vi "test-create-path-trajectory-2.vi"() -> ()   [LabVIEW 2019]
uses:
  <vilib>/Rock Robotics/WPI/ThirdParty/MJansen/PathPlanner/TypeDef/PathPlannerTrajectory.ctl
  <vilib>/Rock Robotics/WPI/ThirdParty/MJansen/PathPlanner/TypeDef/PathPlannerTrajectoryState.ctl
  <vilib>/Rock Robotics/WPI/ThirdParty/JAS_Junk/TrajLib/TypeDef/TRANSLATION2D.ctl
  <vilib>/Rock Robotics/WPI/ThirdParty/JAS_Junk/TrajLib/TypeDef/ROTATION2D.ctl
  <vilib>/Rock Robotics/WPI/ThirdParty/MJansen/PathPlanner/TypeDef/PathPlannerPathConstraints.ctl
  <vilib>/Rock Robotics/WPI/ThirdParty/JAS_Junk/TrajLib/TypeDef/TRAJ_STATE.ctl
  <vilib>/Rock Robotics/WPI/ThirdParty/JAS_Junk/TrajLib/TypeDef/POSE2D.ctl
  <vilib>/Rock Robotics/WPI/ThirdParty/JAS_Junk/TrajLib/TypeDef/CHASSIS_SPEEDS.ctl
  <vilib>/Rock Robotics/WPI/ThirdParty/MJansen/PathPlanner/TypeDef/PathPlannerGoalEndState.ctl
  <vilib>/Rock Robotics/WPI/ThirdParty/MJansen/PathPlanner/TypeDef/PathPlannerPath.ctl
  <vilib>/Rock Robotics/WPI/ThirdParty/MJansen/PathPlanner/TypeDef/PathPlannerRotationTarget.ctl
  <vilib>/Rock Robotics/WPI/ThirdParty/MJansen/PathPlanner/TypeDef/PathPlannerConstraintsZone.ctl
  <vilib>/Rock Robotics/WPI/ThirdParty/MJansen/PathPlanner/TypeDef/PathPlannerEventMarker.ctl
  <vilib>/Rock Robotics/WPI/ThirdParty/MJansen/PathPlanner/TypeDef/PathPlannerCommand.ctl
  <vilib>/Rock Robotics/WPI/ThirdParty/MJansen/PathPlanner/TypeDef/PathPlannerPathPoint.ctl
  <vilib>/Rock Robotics/WPI/ThirdParty/JAS_Junk/TrajLib/Conv_Deg_Radians.vi
  <vilib>/Rock Robotics/WPI/ThirdParty/JAS_Junk/TrajLib/Rotation2d_CreateAngle.vi
  <vilib>/Rock Robotics/WPI/ThirdParty/JAS_Junk/TrajLib/Pose2d_getTranslation.vi
  <vilib>/Rock Robotics/WPI/ThirdParty/JAS_Junk/TrajLib/Translation2d_GetDistance.vi
  <vilib>/Rock Robotics/WPI/ThirdParty/JAS_Junk/TrajLib/Pose2d_getRotation.vi
  <vilib>/Rock Robotics/WPI/ThirdParty/JAS_Junk/TrajLib/Translation2d_Create_DistAng.vi
  <vilib>/Rock Robotics/WPI/ThirdParty/JAS_Junk/TrajLib/Translation2d_Plus.vi
  <vilib>/Rock Robotics/WPI/ThirdParty/JAS_Junk/TrajLib/Rotation2d_Plus.vi
  <vilib>/Rock Robotics/WPI/ThirdParty/JAS_Junk/TrajLib/Util_CalcDist.vi
  <vilib>/Rock Robotics/WPI/ThirdParty/JAS_Junk/TrajLib/Rotation2d_GetAngleCosSin.vi
  <vilib>/Rock Robotics/WPI/ThirdParty/JAS_Junk/TrajLib/Translation2d_Create.vi
  <vilib>/Rock Robotics/WPI/ThirdParty/JAS_Junk/TrajLib/Rotation2d_RotateBy.vi
  <vilib>/Rock Robotics/WPI/ThirdParty/JAS_Junk/TrajLib/Rotation2d_CreateXY.vi
  <vilib>/Rock Robotics/WPI/ThirdParty/MJansen/PathPlanner/PathPlanner24.lvlib
  <vilib>/Rock Robotics/WPI/ThirdParty/JAS_Junk/TrajLib/Trajectory_Library.lvlib
panel:
  in  "Tab Control":T1(tab)
  in  "Position 1":T2={"TRANSLATION"={"X"=1.0, "Y"=1.0}, "ROTATION"={"VALUE"=0.0, "COS"=1.0, "SIN"=0.0}} {"ROTATION"."SIN" format="%13.4f"; "ROTATION"."COS" format="%13.4f"; "ROTATION"."VALUE" format="%13.4f"; "TRANSLATION"."Y" format="%14.3f"; "TRANSLATION"."X" format="%14.3f"}
  in  "Position 2":T2={"TRANSLATION"={"X"=1.3, "Y"=1.0}, "ROTATION"={"VALUE"=0.0, "COS"=1.0, "SIN"=0.0}} {"ROTATION"."SIN" format="%13.4f"; "ROTATION"."COS" format="%13.4f"; "ROTATION"."VALUE" format="%13.4f"; "TRANSLATION"."Y" format="%14.3f"; "TRANSLATION"."X" format="%14.3f"}
  in  "Position 3":T2={"TRANSLATION"={"X"=4.0, "Y"=3.7}, "ROTATION"={"VALUE"=1.57, "COS"=0.0, "SIN"=1.0}} {"ROTATION"."SIN" format="%13.4f"; "ROTATION"."COS" format="%13.4f"; "ROTATION"."VALUE" format="%13.4f"; "TRANSLATION"."Y" format="%14.3f"; "TRANSLATION"."X" format="%14.3f"}
  in  "Position 4":T2={"TRANSLATION"={"X"=4.0, "Y"=4.0}, "ROTATION"={"VALUE"=1.57, "COS"=0.0, "SIN"=1.0}} {"ROTATION"."SIN" format="%13.4f"; "ROTATION"."COS" format="%13.4f"; "ROTATION"."VALUE" format="%13.4f"; "TRANSLATION"."Y" format="%14.3f"; "TRANSLATION"."X" format="%14.3f"}
  in  "stop":bool
  in  "StartingSpeeds":T5 {"vOmega" format="%10.3f"; "vY" format="%10.3f"; "vX" format="%10.3f"}
  out "Error":bool
  out "Error 2":bool
  out "Bezier":T3[](array[typedef]) {"Y" format="%14.3f"; "X" format="%14.3f"}
  out "PathPlannerConstraints":T6
  out "GoalEndState":T7={"Velocity"=0.0, "Rotation"={"VALUE"=0.0, "COS"=1.0, "SIN"=0.0}} {"Rotation"."SIN" format="%13.4f"; "Rotation"."COS" format="%13.4f"; "Rotation"."VALUE" format="%13.4f"}
  in  "Angle_Degrees":dbl=90.0
  in  "Velocity":dbl format="%#_13g"
  out "PathPlannerPath":T8={"BezierPoints"=[], "PreviewStartingRotation"={"VALUE"=0.0, "COS"=1.0, "SIN"=0.0}, "Reversed"=FALSE, "RotationTargets"=[], "ConstraintZones"=[], "EventMarkers"=[], "GlobalConstraints"={"MaxVelocityMps;"=0.0, "MaxAccelerationMpsSq;"=0.0, "MaxAngularVelRadPsEc;"=0.0, "MaxAngularAccRadPSecSq"=0.0, "Exists"=FALSE}, "GoalEndState"={"Velocity"=0.0, "Rotation"={"VALUE"=0.0, "COS"=1.0, "SIN"=0.0}}, "AllPoints"=[]} {"AllPoints"."HolonomicRotation"."SIN" format="%13.4f"; "AllPoints"."HolonomicRotation"."COS" format="%13.4f"; "AllPoints"."HolonomicRotation"."VALUE" format="%13.4f"; "AllPoints"."Position"."Y" format="%14.3f"; "AllPoints"."Position"."X" format="%14.3f"; "GoalEndState"."Rotation"."SIN" format="%13.4f"; "GoalEndState"."Rotation"."COS" format="%13.4f"; "GoalEndState"."Rotation"."VALUE" format="%13.4f"; "EventMarkers"."lastRobotPos"."Y" format="%14.3f"; "EventMarkers"."lastRobotPos"."X" format="%14.3f"; "EventMarkers"."markerPos"."Y" format="%14.3f"; "EventMarkers"."markerPos"."X" format="%14.3f"; "RotationTargets"."target"."SIN" format="%13.4f"; "RotationTargets"."target"."COS" format="%13.4f"; "RotationTargets"."target"."VALUE" format="%13.4f"; "PreviewStartingRotation"."SIN" format="%13.4f"; "PreviewStartingRotation"."COS" format="%13.4f"; "PreviewStartingRotation"."VALUE" format="%13.4f"; "BezierPoints"."Y" format="%14.3f"; "BezierPoints"."X" format="%14.3f"}
  out "PathPlannerTrajectory":T14 {"States"."TargetHolonomicRotation"."SIN" format="%13.4f"; "States"."TargetHolonomicRotation"."COS" format="%13.4f"; "States"."TargetHolonomicRotation"."VALUE" format="%13.4f"; "States"."Heading"."SIN" format="%13.4f"; "States"."Heading"."COS" format="%13.4f"; "States"."Heading"."VALUE" format="%13.4f"; "States"."PositionMeters"."Y" format="%14.3f"; "States"."PositionMeters"."X" format="%14.3f"}
  out "outPathPlannerStates":T15[](array[typedef]) {"TargetHolonomicRotation"."SIN" format="%13.4f"; "TargetHolonomicRotation"."COS" format="%13.4f"; "TargetHolonomicRotation"."VALUE" format="%13.4f"; "Heading"."SIN" format="%13.4f"; "Heading"."COS" format="%13.4f"; "Heading"."VALUE" format="%13.4f"; "PositionMeters"."Y" format="%14.3f"; "PositionMeters"."X" format="%14.3f"}
  in  "Down Button":bool
  in  "Up Button":bool
  in  "index":i32 step=20
  out "LabVIEWStateCount":i32
  out "LabVIEWStates":T16[](array[typedef]) {"POSE"."ROTATION"."SIN" format="%13.4f"; "POSE"."ROTATION"."COS" format="%13.4f"; "POSE"."ROTATION"."VALUE" format="%13.4f"; "POSE"."TRANSLATION"."Y" format="%14.3f"; "POSE"."TRANSLATION"."X" format="%14.3f"}
  out "XY SPLINE":cluster{dbl[], dbl[]}[](graph)
  out "XY Graph":cluster{dbl[], dbl[]}[](graph)
  out "Sample Graph":dbl[][](graph)
  out "LabVIEW Time Plot":cluster{dbl[], dbl[]}[](graph)
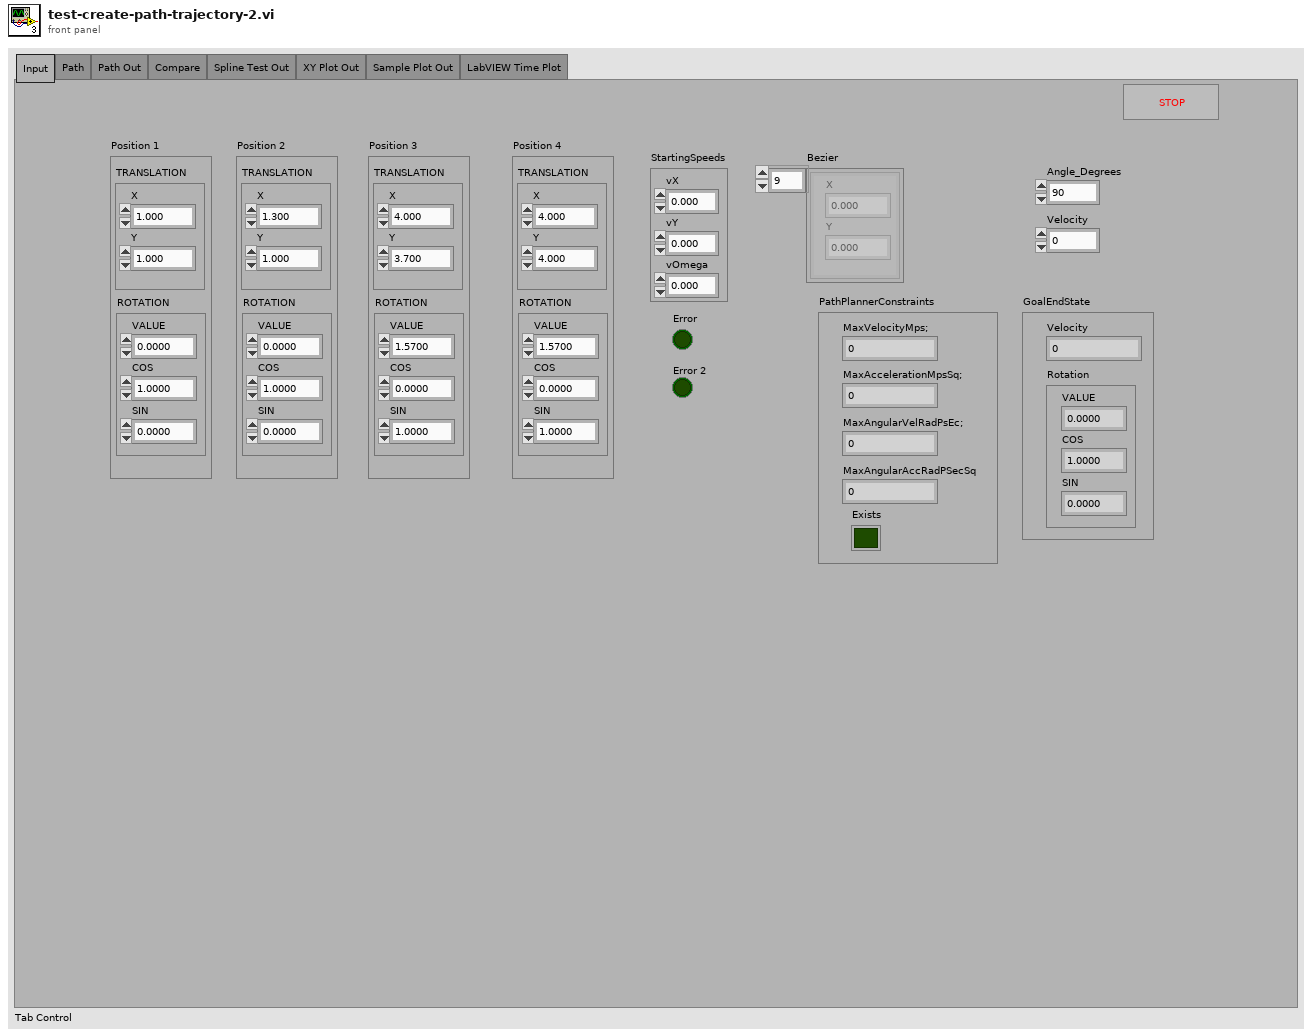
[diagram p1: front panel]
types:
  T1 = enum32{"Input", "Path", "Path Out", "Compare", "Spline Test Out", "XY Plot Out", "Sample Plot Out", "LabVIEW Time Plot"}
  T2 = typedef "Trajectory_Library.lvlib/POSE2D.ctl" = cluster{"TRANSLATION":T3, "ROTATION":T4}
  T3 = typedef "Trajectory_Library.lvlib/TRANSLATION2D.ctl" = cluster{"X":dbl, "Y":dbl}
  T4 = typedef "Trajectory_Library.lvlib/ROTATION2D.ctl" = cluster{"VALUE":dbl, "COS":dbl, "SIN":dbl}
  T5 = typedef "Trajectory_Library.lvlib/CHASSIS_SPEEDS.ctl" = cluster{"vX":dbl, "vY":dbl, "vOmega":dbl}
  T6 = typedef "PathPlanner24.lvlib/PathPlannerPathConstraints.ctl" = cluster{"MaxVelocityMps;":dbl, "MaxAccelerationMpsSq;":dbl, "MaxAngularVelRadPsEc;":dbl, "MaxAngularAccRadPSecSq":dbl, "Exists":bool}
  T7 = typedef "PathPlanner24.lvlib/PathPlannerGoalEndState.ctl" = cluster{"Velocity":dbl, "Rotation":T4}
  T8 = typedef "PathPlanner24.lvlib/PathPlannerPath.ctl" = cluster{"BezierPoints":T3[], "PreviewStartingRotation":T4, "Reversed":bool, "RotationTargets":T9[], "ConstraintZones":T10[], "EventMarkers":T11[], "GlobalConstraints":T6, "GoalEndState":T7, "AllPoints":T13[]}
  T9 = typedef "PathPlanner24.lvlib/PathPlannerRotationTarget.ctl" = cluster{"target":T4, "WaypointRelativePosition":dbl, "Exists":bool}
  T10 = typedef "PathPlanner24.lvlib/PathPlannerConstraintsZone.ctl" = cluster{"minWaypointPos":dbl, "maxWaypointPos":dbl, "Constraints":T6, "Present":bool}
  T11 = typedef "PathPlanner24.lvlib/PathPlannerEventMarker.ctl" = cluster{"WaypointRelativePos":dbl, "minimumTriggerDistance":dbl, "markerPos":T3, "lastRobotPos":T3, "Command":T12}
  T12 = typedef "PathPlanner24.lvlib/PathPlannerCommand.ctl" = cluster{"waitTime":dbl, "name":string, "type":string, "pathName":string, "commands":cluster{"type":string, "waitTime":dbl, "name":string, "pathName":string}[]}
  T13 = typedef "PathPlanner24.lvlib/PathPlannerPathPoint.ctl" = cluster{"Position":T3, "HolonomicRotation":T4, "DistAlongPath":dbl, "CurveRadius":dbl, "MaxV":dbl, "Constraints":T6, "HolonomicRotationExists":bool}
  T14 = typedef "PathPlanner24.lvlib/PathPlannerTrajectory.ctl" = cluster{"States":T15[]}
  T15 = typedef "PathPlanner24.lvlib/PathPlannerTrajectoryState.ctl" = cluster{"TimeSeconds":dbl, "VelocityMPS":dbl, "AccerationMpsSq":dbl, "HeadingAngularVelRadPerSec":dbl, "PositionMeters":T3, "Heading":T4, "TargetHolonomicRotation":T4, "CurvatureRadPerMeter":dbl, "DeltaPos":dbl, "PathPlannerConstraints":T6}
  T16 = typedef "Trajectory_Library.lvlib/TRAJ_STATE.ctl" = cluster{"TimeSeconds":dbl, "Velocity":dbl, "Acceleration":dbl, "POSE":T2, "Curvature":dbl}
  T17 = typedef "Trajectory_Library.lvlib/TRAJECTORY.ctl" = cluster{"TotalTImeSecs":dbl, "States":T16[]}
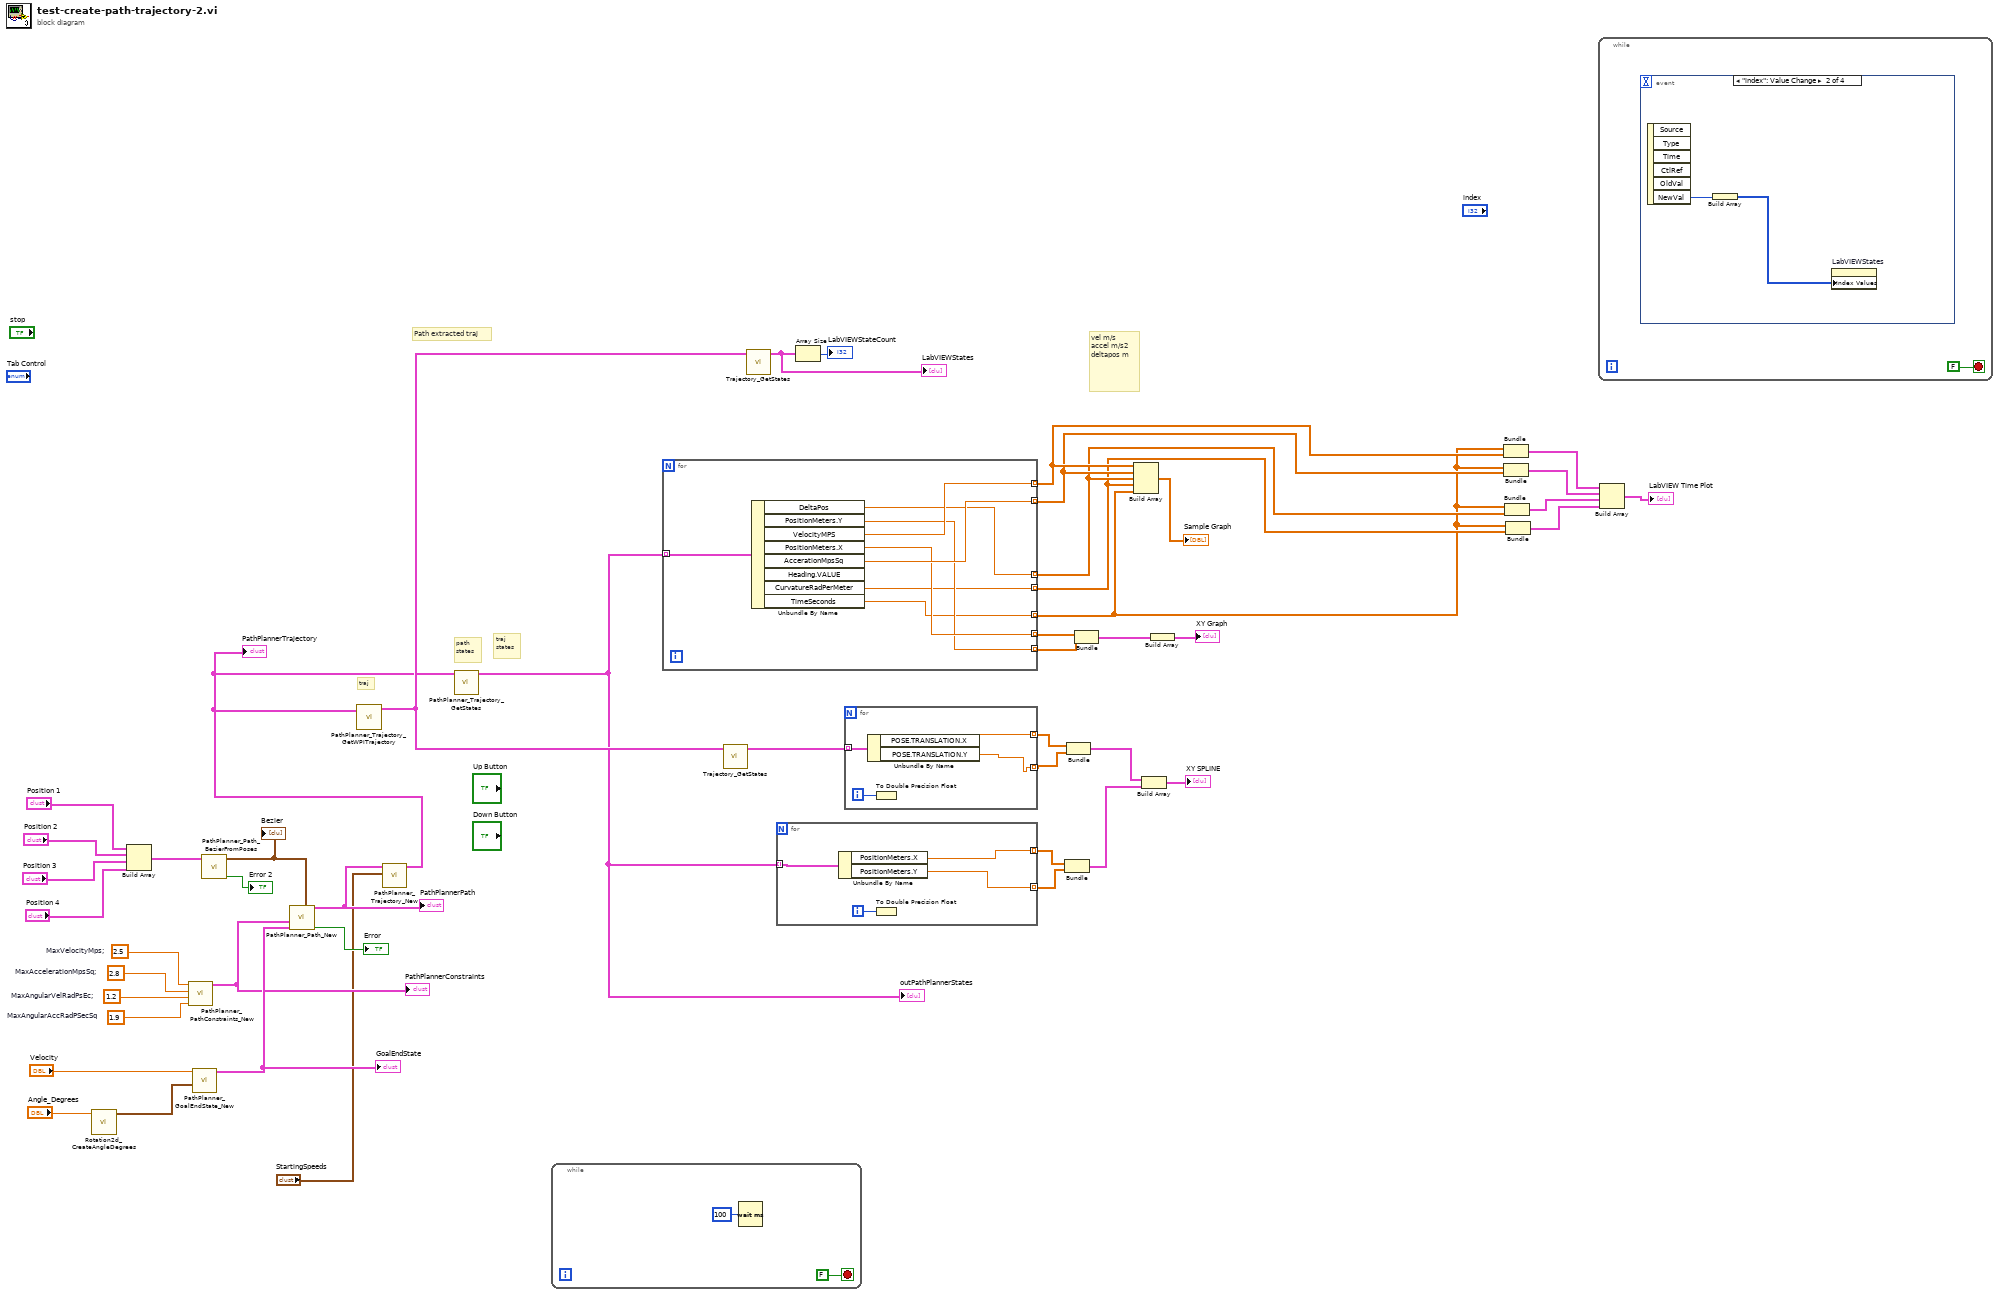
[diagram p0: block diagram]
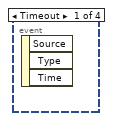
[diagram p2: hidden frame]
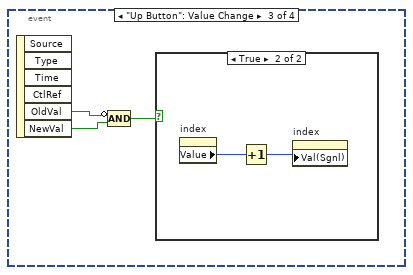
[diagram p3: hidden frame]
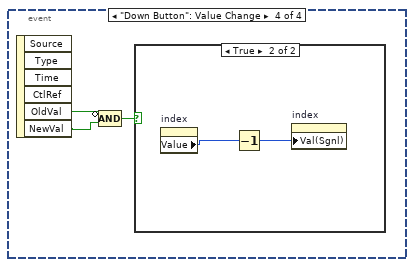
[diagram p5: hidden frame]
diagram:
  w10 = 2.5  # MaxVelocityMps;
  w11 = 2.8  # MaxAccelerationMpsSq;
  w12 = 1.2  # MaxAngularVelRadPsEc;
  w9 = 1.9  # MaxAngularAccRadPSecSq
  # "vel m/s\naccel m/s2\ndeltapos m"
  # "Path extracted traj"
  # "traj"
  # "traj\nstates"
  # "path\nstates"
  n1 = call <vilib>:"Rotation2d_CreateAngleDegrees.vi"("Angle_Degrees"="Angle_Degrees") -> ("ROTATION"=w1:T4)  [unwired: 10 in]
  n2 = Build Array("Position 1", "Position 2", "Position 3", "Position 4") -> (w16:T2[])
  n3 = call <vilib>:"PathPlanner_PathConstraints_New.vi"("MaxAngularAccRadPSecSq"=w9, "MaxAngularVelRadPsEc;"=w12, "MaxAccelerationMpsSq;"=w11, "MaxVelocityMps;"=w10) -> ("PathPlannerConstraints"=w13:T6)  [unwired: 7 in]
  "PathPlannerConstraints" <- w13
  n4 = call <vilib>:"PathPlanner_GoalEndState_New.vi"("Rotation"=w1, "Velocity"="Velocity") -> ("GoalEndState"=w14:T7)  [unwired: 9 in]
  "GoalEndState" <- w14
  n5 = call <vilib>:"PathPlanner_Path_BezierFromPoses.vi"("Poses"=w16) -> ("Error"=→"Error 2":bool, "Bezier"=w15:T3[])  [unwired: 9 in]
  "Bezier" <- w15
  n6 = call <vilib>:"PathPlanner_Path_New.vi"("BezierPoints"=w15, "GoalEndState"=w14, "GlobalConstraints"=w13) -> ("Error"=→"Error":bool, "PathPlannerPath"=w6:T8)  [unwired: 7 in]
  "PathPlannerPath" <- w6
  n7 = call <vilib>:"PathPlanner_Trajectory_New.vi"("StartingSpeeds"="StartingSpeeds", "Path"=w6) -> ("PathPlannerTrajectory"=w5:T14)  [unwired: 9 in]
  "PathPlannerTrajectory" <- w5
  n8 = call <vilib>:"PathPlanner_Trajectory_GetWPITrajectory.vi"("PathPlannerTrajectory"=w5) -> ("TRAJECTORY"=w34:T17)  [unwired: 9 in, 1 out]
  n9 = call <vilib>:"PathPlanner_Trajectory_GetStates.vi"("PathPlannerTrajectory"=w5) -> ("PathPlannerStates"=w31:T15[])  [unwired: 10 in]
  "outPathPlannerStates" <- w31
  n10 = while {
    stop <- FALSE stop-if-true
    n11 = Wait (ms)(milliseconds to wait=u32 100) -> ()  [unwired: 1 out]
  }
  n12 = for {
    tunnel: [w57] -> w29 mode=indexing
    tunnel: [w56] -> w28 mode=indexing
    tunnel: [w51] -> w27 mode=indexing
    tunnel: [w55] -> w46 mode=indexing
    tunnel: [w54] -> w45 mode=indexing
    tunnel: w31 -> [w53] mode=indexing
    tunnel: [w52] -> w26 mode=indexing
    tunnel: [w50] -> w21 mode=indexing
    n13 = Unbundle By Name(w53) -> ("DeltaPos"=w51:dbl, "PositionMeters.Y"=w54:dbl, "VelocityMPS"=w57:dbl, "PositionMeters.X"=w55:dbl, "AccerationMpsSq"=w56:dbl, "CurvatureRadPerMeter"=w52:dbl, "TimeSeconds"=w50:dbl)  [unwired: 1 out]
  }
  n14 = call <vilib>:"Trajectory_GetStates.vi"("TRAJECTORY"=w34) -> ("States"=w35:T16[])  [unwired: 10 in]
  n15 = call <vilib>:"Trajectory_GetStates.vi"("TRAJECTORY"=w34) -> ("States"=w32:T16[])  [unwired: 10 in]
  "LabVIEWStates" <- w32
  n16 = for {
    tunnel: [w60] -> w40 mode=indexing
    tunnel: w31 -> [w59] mode=indexing
    tunnel: [w58] -> w39 mode=indexing
    i -> [w61]
    n17 = Unbundle By Name(w59) -> ("PositionMeters.X"=w60:dbl, "PositionMeters.Y"=w58:dbl)
    n18 = To Double Precision Float(number=w61) -> ()  [unwired: 1 out]
  }
  n19 = Array Size(array=w32) -> (size(s)=→"LabVIEWStateCount":i32)
  n20 = for {
    tunnel: [w64] -> w42 mode=indexing
    tunnel: [w63] -> w41 mode=indexing
    tunnel: w35 -> [w62] mode=indexing
    i -> [w65]
    n21 = Unbundle By Name(w62) -> ("POSE.TRANSLATION.X"=w64:dbl, "POSE.TRANSLATION.Y"=w63:dbl)
    n22 = To Double Precision Float(number=w65) -> ()  [unwired: 1 out]
  }
  n23 = Bundle(w40, w39) -> (w37:cluster{dbl[], dbl[]})  [unwired: 1 in]
  n24 = Bundle(w42, w41) -> (w38:cluster{dbl[], dbl[]})  [unwired: 1 in]
  n25 = Bundle(w46, w45) -> (w44:cluster{dbl[], dbl[]})  [unwired: 1 in]
  n26 = Build Array(w29, w28, w27, w26, w21) -> (→"Sample Graph":dbl[][])
  n27 = Build Array(w38, w37) -> (→"XY SPLINE":cluster{dbl[], dbl[]}[])
  n28 = Build Array(w44) -> (→"XY Graph":cluster{dbl[], dbl[]}[])
  n29 = Bundle(w21, w29) -> (w25:cluster{dbl[], dbl[]})  [unwired: 1 in]
  n30 = Bundle(w21, w28) -> (w24:cluster{dbl[], dbl[]})  [unwired: 1 in]
  n31 = Bundle(w21, w27) -> (w23:cluster{dbl[], dbl[]})  [unwired: 1 in]
  n32 = Bundle(w21, w26) -> (w22:cluster{dbl[], dbl[]})  [unwired: 1 in]
  n33 = while {
    stop <- FALSE stop-if-true
    n34 = event shown="[1] \"index\": Value Change" {
      selector: _ -> [_ _ _ _]
      dyn-events: _ -> [_ _ _ _]
      timeout: _ -> [_ _ _ _]
      event Timeout {
        n35 = event-data() -> ()  [unwired: 1 in, 3 out]
      }
      event "index": Value Change {
        n36 = event-data() -> ("NewVal"=w68:i32)  [unwired: 1 in, 5 out]
        n37 = Build Array(w68) -> (w67:i32[])
        n38 = property on="LabVIEWStates" class="Arr (strict)"("Index Values"=w67) -> ()  [unwired: 2 in, 2 out]
      }
      event "Up Button": Value Change {
        n39 = event-data() -> ("OldVal"=w71:bool, "NewVal"=w70:bool)  [unwired: 1 in, 4 out]
        n40 = Compound Arithmetic op=AND(invert w71, w70) -> (w69:bool)
        n41 = case shown="True" w69 {
          frame False {
          }
          frame True {
            n42 = property on="index" class="DigNum (strict)"() -> ("Value"=w72:i32)  [unwired: 2 in, 2 out]
            n43 = Increment(x=w72) -> (x+1=w73:i32)
            n44 = property on="index" class="DigNum (strict)"("Val(Sgnl)"=w73) -> ()  [unwired: 2 in, 2 out]
          }
        }
      }
      event "Down Button": Value Change {
        n45 = event-data() -> ("OldVal"=w75:bool, "NewVal"=w74:bool)  [unwired: 1 in, 4 out]
        n46 = Compound Arithmetic op=AND(invert w75, w74) -> (w76:bool)
        n47 = case shown="True" w76 {
          frame False {
          }
          frame True {
            n48 = property on="index" class="DigNum (strict)"() -> ("Value"=w77:i32)  [unwired: 2 in, 2 out]
            n49 = Decrement(x=w77) -> (x-1=w78:i32)
            n50 = property on="index" class="DigNum (strict)"("Val(Sgnl)"=w78) -> ()  [unwired: 2 in, 2 out]
          }
        }
      }
    }
  }
  n51 = Build Array(w25, w24, w23, w22) -> (→"LabVIEW Time Plot":cluster{dbl[], dbl[]}[])
